vi "Replace ID with Alias.vi"(1 "Message Log Data":string[](array[string])) -> (0 "Message Log Data (Short IDs)":string[](array[string]))   [LabVIEW 2017, in "Message Log.lvclass"]
uses:
  Message Log.lvclass
  <vilib>/addons/_Workers/Library/Workers.lvlib
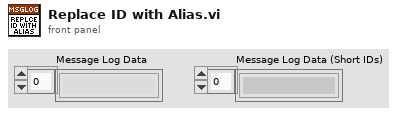
[diagram p1: front panel]
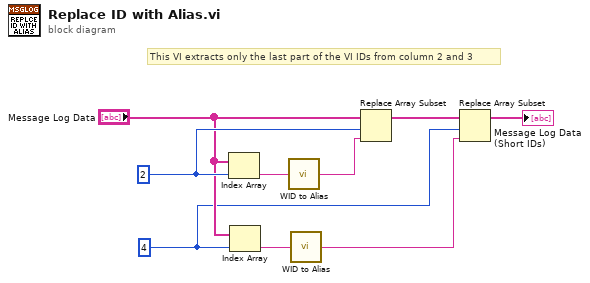
[diagram p0: block diagram]
diagram:
  w4 = 4 ("index")
  w8 = 2 ("index")
  # "This VI extracts only the last part of the VI IDs from column 2 and 3"
  n1 = Index Array(array="Message Log Data", index=w8) -> (element=w9:string)
  n2 = Index Array(array="Message Log Data", index=w4) -> (element=w7:string)
  n3 = call <vilib>:"WID to Alias.vi"("WID"=w9) -> ("Alias"=w2:string)
  n4 = call <vilib>:"WID to Alias.vi"("WID"=w7) -> ("Alias"=w1:string)
  n5 = Replace Array Subset(array="Message Log Data", new element=w2, index=w8) -> (w5:string[])
  n6 = Replace Array Subset(array=w5, new element=w1, index=w4) -> (→"Message Log Data (Short IDs)":string[])
